vi "RSZVB Set Generator Port Resolution Bandwidth.vi"(7 "Generator Port (1)":i32=1, 8 "error in (no error)":errorcluster {"code" format="%.0x"}, 9 "Resolution Bandwidth (30.0e6 Hz)":dbl=10000.0 min=1.0 max=30000000.0 format="%^.3e", 10 "Channel (1)":i32=1, 11 "VISA session":refnum<visa-resource-name>) -> (0 "error out":errorcluster {"code" format="%.0x"}, 3 "dup VISA session":refnum<visa-resource-name>)   [LabVIEW 2011]
doc: "Defines the resolution bandwidth of the analyzer for all partial measurements where an external generator <Gen> is used as a source.\n\nRemote-control command(s):\n[SENSe<Ch>:]BANDwidth|BWIDth[:RESolution]:GENerator<Gen>"
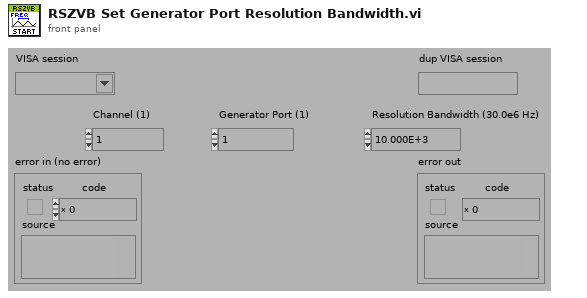
[diagram p1: front panel]
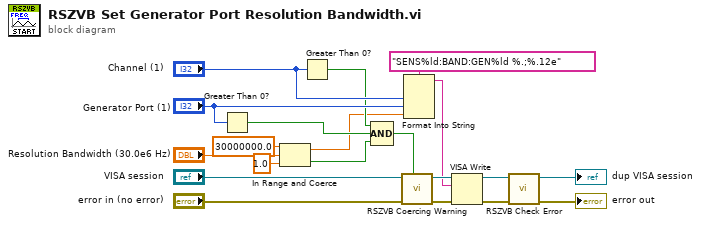
[diagram p0: block diagram]
diagram:
  n1 = Greater Than 0?(x="Generator Port (1)") -> (x > 0?=w7:bool)
  n2 = In Range and Coerce(upper limit=30000000.0, x="Resolution Bandwidth (30.0e6 Hz)", lower limit=1.0) -> (coerced(x)=w3:dbl, In Range?=w4:bool)
  n3 = Greater Than 0?(x="Channel (1)") -> (x > 0?=w8:bool)
  n4 = Compound Arithmetic op=AND(w8, w7, w4) -> (w6:bool)
  n5 = call "RSZVB Coercing Warning.vi"("In Range?"=w6, "error in (no error)"="error in (no error)", "VISA session"="VISA session") -> ("error out"=w18:errorcluster, "dup VISA session"=w19:refnum<visa-resource-name>)  [unwired: 7 in]
  n6 = Format Into String(format string="SENS%ld:BAND:GEN%ld %.;%.12e", "Channel (1)", "Generator Port (1)", w3) -> (resulting string=w15:string)  [unwired: 2 in, 1 out]
  n7 = VISA Write(VISA resource name=w19, write buffer=w15, error in (no error)=w18) -> (VISA resource name out=w16:refnum<visa-resource-name>, error out=w17:errorcluster)  [unwired: 1 out]
  n8 = call "RSZVB Check Error.vi"("error in (no error)"=w17, "VISA session"=w16) -> ("error out"=→"error out":errorcluster, "dup VISA session"=→"dup VISA session":refnum<visa-resource-name>)  [unwired: 8 in]
